vi "test_DeviceManager_StartICL.vi"(8 "error in":errorcluster) -> (0 "error out":errorcluster)   [LabVIEW 2023, in "horiba.test.lvlib"]
doc: "_____\nCreated using DQMH Event Scripter 7.0.0.1280."
uses:
  <vilib>/addons/_JKI Toolkits/Caraya/classes/Assert/Assert Not Error.vi
  <vilib>/addons/_JKI Toolkits/Caraya/classes/Assert/Assert True.vi
  horiba.test.lvlib
  Classes/DeviceManager/DeviceManager.lvlib
  <vilib>/addons/_JKI Toolkits/Caraya/classes/Assert/Assert.lvclass
  <vilib>/addons/_JKI Toolkits/Caraya/classes/Test/Test.lvclass
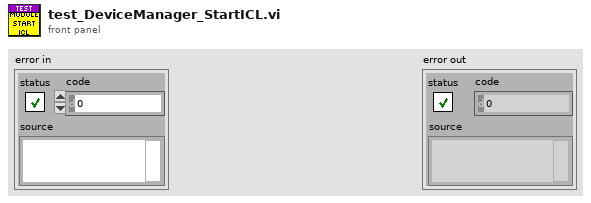
[diagram p1: front panel]
types:
  T1 = typedef "horiba.lvlib/DeviceManager.lvlib/Broadcast Events--cluster.ctl" = cluster{"Module Did Init":refnum<user-event>, "Status Updated":refnum<user-event>, "Error Reported":refnum<user-event>, "Module Did Stop":refnum<user-event>, "Update Module Execution Status":refnum<user-event>, "iclIsRunning":refnum<user-event>, "websocketConnectionOpened":refnum<user-event>, "devicesDiscovered":refnum<user-event>}
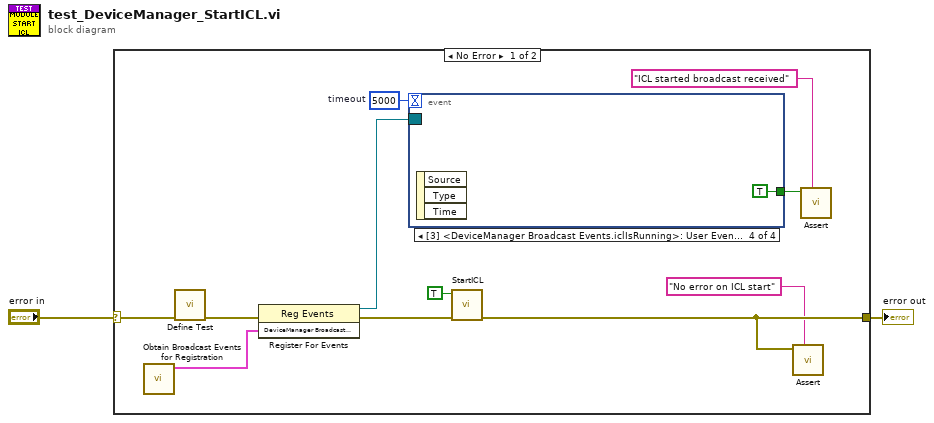
[diagram p0: block diagram]
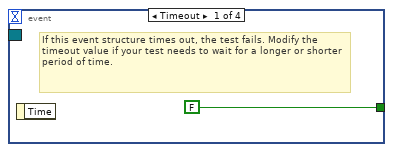
[diagram p2: hidden frame]
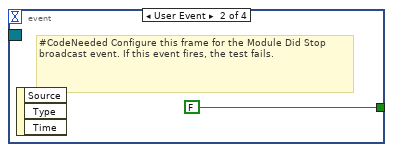
[diagram p3: hidden frame]
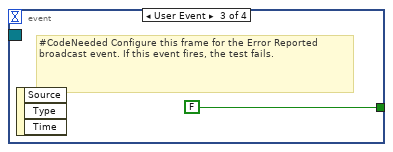
[diagram p4: hidden frame]
diagram:
  n1 = case shown="No Error" "error in" {
    selector: "error in" -> [w13 w18]
    tunnel: [w7 w18] -> w1
    frame No Error {
      w9 = 5000  # timeout
      n2 = call "Obtain Broadcast Events for Registration.vi"() -> ("DeviceManager Broadcast Events"=w11:T1)  [unwired: 9 in, 2 out]
      n3 = call <vilib>:"Define Test.vi"("error in (no error)"=w13) -> ("error out"=w6:errorcluster)  [unwired: 9 in, 1 out]
      n4 = register-events(error in=w6, w11) -> (reference out=w10:refnum<event-registration>, error out=w12:errorcluster)  [unwired: 1 in]
      n5 = event shown="[3] <DeviceManager Broadcast Events.iclIsRunning>: User Event" {
        selector: w10 -> [_ _ _ _]
        dyn-events: _ -> [_ _ _ _]
        timeout: w9 -> [_ _ _ _]
        tunnel: [FALSE FALSE FALSE TRUE] -> w8
        event Timeout {
          # "If this event structure times out, the test fails. Modify the timeout value if your test needs to wait for a longer or shorter period of time."
          n6 = event-data() -> ()  [unwired: 1 in, 1 out]
        }
        event User Event {
          # "#CodeNeeded Configure this frame for the Module Did Stop broadcast event. If this event fires, the test fails."
          n7 = event-data() -> ()  [unwired: 1 in, 3 out]
        }
        event User Event {
          # "#CodeNeeded Configure this frame for the Error Reported broadcast event. If this event fires, the test fails."
          n8 = event-data() -> ()  [unwired: 1 in, 3 out]
        }
        event User Event {
          n9 = event-data() -> ()  [unwired: 1 in, 3 out]
        }
      }
      n10 = call "StartICL.vi"("error in"=w12, "show ICL for debugging"=TRUE) -> ("error out"=w7:errorcluster)  [unwired: 9 in]
      n11 = call-poly <vilib>:"Assert.vi"("Label"="No error on ICL start", "Not Error?"=w7) -> ()  [unwired: 8 in, 2 out]
      n12 = call-poly <vilib>:"Assert.vi"("Label"="ICL started broadcast received", "True?"=w8) -> ()  [unwired: 8 in, 2 out]
    }
    frame Error {
    }
  }
  "error out" <- w1
